vi "SubVI_DisabledCode_auto.vi"() -> (3 "Yaw":dbl)   [LabVIEW 2017]
uses:
  <vilib>/Rock Robotics/WPI/ThirdParty/Sensors/navX/_TypeDefs/Z900_navX_ActionTypeDef.ctl
  <vilib>/Rock Robotics/WPI/ThirdParty/Sensors/navX/_TypeDefs/FRIC_navX_DeviceNumbersTypeDef.ctl
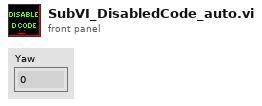
[diagram p1: front panel]
types:
  T1 = typedef "FRIC_navX_DeviceNumbersTypeDef.ctl" = enum16{"Dev0", "Dev1", "Dev2", "Dev3"}
  T2 = typedef "Z900_navX_ActionTypeDef.ctl" = enum16{"None", "Halt", "Normal Read", "Update Serial Protocol", "Update Rate Htz", "Zero-Yaw", "Zero-Displacement", "Zero-Velocity"}
  T3 = cluster{"Yaw":dbl, "Roll":dbl, "Pitch":dbl, "Heading":dbl, "Fused Heading":dbl}
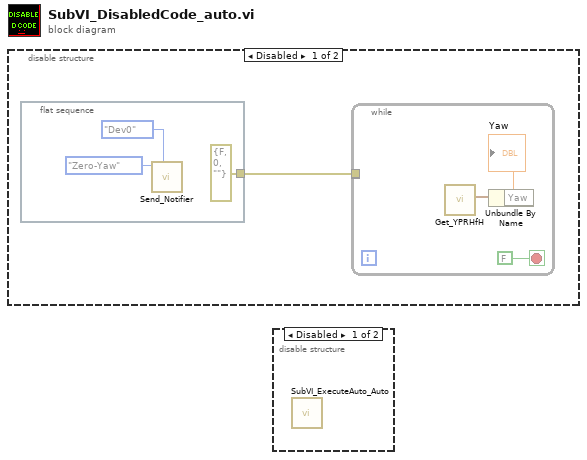
[diagram p0: block diagram]
diagram:
  n1 = disable-structure shown="Disabled" {
    frame Disabled {
      n2 = flat-sequence {
        tunnel: [errorcluster {"status"=FALSE, "code"=0, "source"=""} ("error constant")] -> w1
        frame #0 {
          n3 = call <vilib>:"Send_Notifier.vi"("Device Number"=FRIC_navX_DeviceNumbersTypeDef."Dev0", "navX Action"=Z900_navX_ActionTypeDef."Zero-Yaw") -> ()  [unwired: 10 in]
        }
      }
      n4 = while {
        tunnel: [w2] -> _
        tunnel: w1 -> [w2]
        stop <- FALSE stop-if-true
        n5 = call <vilib>:"Get_YPRHfH.vi"() -> ("YRPHfH"=w5:T3)  [unwired: 11 in]
        n6 = Unbundle By Name(w5) -> ("Yaw"=→"Yaw":dbl)
      }
    }
    frame Enabled {
    }
  }
  n7 = disable-structure shown="Disabled" {
    frame Disabled {
      n8 = call "SubVI_ExecuteAuto_Auto.vi"() -> ()  [unwired: 10 in, 2 out]
    }
    frame Enabled {
    }
  }
